vi "Configure DC Voltage Ratio.vi"(0 "VISA resource name":refnum<visa-resource-name>, 1 "Aperture Seconds":dbl, 2 "Auto Sense Range? (T: Auto)":bool=TRUE, 5 "Auto Range? (T: Auto)":bool, 7 "Manual Range":dbl=1.0, 9 "Set Aperture or NPLC":bool=TRUE, 11 "error in (no error)":errorcluster, 12 "NPLC":dbl=1.0, 13 "Sense Range":u16(ring)=2 items=["0.01", "1", "10"]) -> (4 "VISA resource name out":refnum<visa-resource-name>, 15 "error out":errorcluster)   [LabVIEW 2021, in "Keithley DMM7510.lvlib"]
doc: "This VI configures the DC Voltage ratio measurement and the related parameters."
uses:
  Keithley DMM7510.lvlib
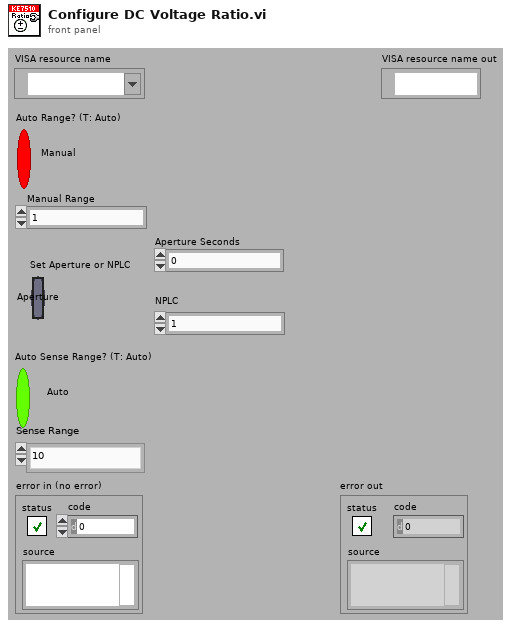
[diagram p1: front panel]
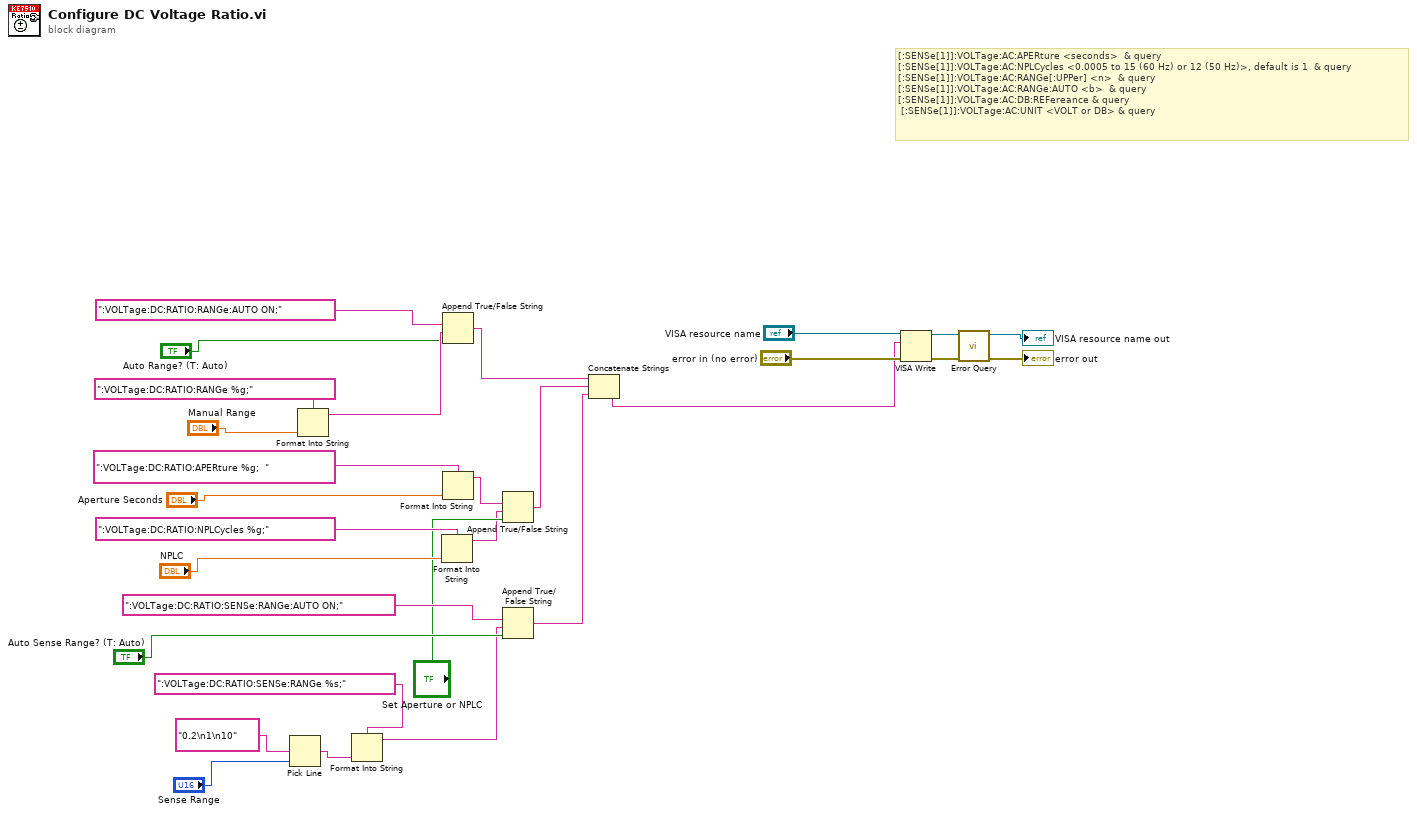
[diagram p0: block diagram]
diagram:
  # "[:SENSe[1]]:VOLTage:AC:APERture <seconds>  & query\n[:SENSe[1]]:VOLTage:AC:NPLCycles <0.0005 to 15 (60 Hz) or 12 (50 Hz)>, default is 1  & query\n[:SENSe[1]]:VOLTage:AC:RANGe[:UPPer] <n>  & query\n[:SENSe[1]]:VOLTage:AC:RANGe:AUTO <b>  & query\n[:SENSe[1]]:VOLTage:AC:DB:REFereance & query\n [:SENSe[1]]:VOLTage:AC:UNIT <VOLT or DB> & query"
  n1 = Pick Line(multi-line string="0.2\n1\n10", line index="Sense Range") -> (output string=w10:string)  [unwired: 1 in]
  n2 = Format Into String(format string=":VOLTage:DC:RATIO:RANGe %g;", "Manual Range") -> (resulting string=w25:string)  [unwired: 2 in, 1 out]
  n3 = Format Into String(format string=":VOLTage:DC:RATIO:SENSe:RANGe %s;", w10) -> (resulting string=w8:string)  [unwired: 2 in, 1 out]
  n4 = Format Into String(format string=":VOLTage:DC:RATIO:NPLCycles %g;", "NPLC") -> (resulting string=w3:string)  [unwired: 2 in, 1 out]
  n5 = Append True/False String(1:"Auto Range? (T: Auto)", 2:w25, 3:":VOLTage:DC:RATIO:RANGe:AUTO ON;") -> (0:w22:string)  [unwired: 1 in]
  n6 = Format Into String(format string=":VOLTage:DC:RATIO:APERture %g;  ", "Aperture Seconds") -> (resulting string=w2:string)  [unwired: 2 in, 1 out]
  n7 = Append True/False String(1:"Set Aperture or NPLC", 2:w3, 3:w2) -> (0:w1:string)  [unwired: 1 in]
  n8 = Append True/False String(1:"Auto Sense Range? (T: Auto)", 2:w8, 3:":VOLTage:DC:RATIO:SENSe:RANGe:AUTO ON;") -> (0:w7:string)  [unwired: 1 in]
  n9 = Concatenate Strings(w22, w1, w7) -> (w21:string)
  n10 = VISA Write(VISA resource name="VISA resource name", write buffer=w21, error in (no error)="error in (no error)") -> (VISA resource name out=w20:refnum<visa-resource-name>, error out=w19:errorcluster)  [unwired: 1 out]
  n11 = call "Error Query.vi"("error in (no error)"=w19, "VISA resource name"=w20) -> ("error out"=→"error out":errorcluster, "VISA resource name out"=→"VISA resource name out":refnum<visa-resource-name>)  [unwired: 6 in, 2 out]
